vi "Get Double Message.vi"(8 "error in (no error)":errorcluster, 11 "Message Double in":refnum<class "Message Double.lvclass">) -> (0 "error out":errorcluster, 1 "Value":dbl, 2 "Name":string, 3 "Message Double out":refnum<class "Message Double.lvclass">)   [LabVIEW 2016, in "Stream Mediator.lvlib" / "Message Double.lvclass"]
doc: "--\nCopyright © 2017 Composed SystemsI All rights reserved.\n\nAuthor: Jon McBee <jon.mcbee@composed.io>\n\nThis library is provided \"AS IS\" ,WITHOUT WARRANTIES OR\nCONDITIONS OF ANY KIND, either express or implied.\n\nComposed Systems -- composed.io\n\nStream 0.0.1.1\nJon McBee - Composed Systems\nCopyright (c) 2017, Composed Systems"
uses:
  <userlib>/Composed Systems/Stream/Mediator/Classes/Message Double/Message Double.lvclass
  C:/Program Files (x86)/National Instruments/LabVIEW 2016/user.lib/Composed Systems/Stream/Mediator/Classes/Message Interface/Message Interface.lvclass
  <userlib>/Composed Systems/Stream/Mediator/Classes/Message Double/Message Double.lvclass/Message Double.ctl
  <userlib>/Composed Systems/Stream/Mediator/Classes/Message Interface/Message Interface.lvclass
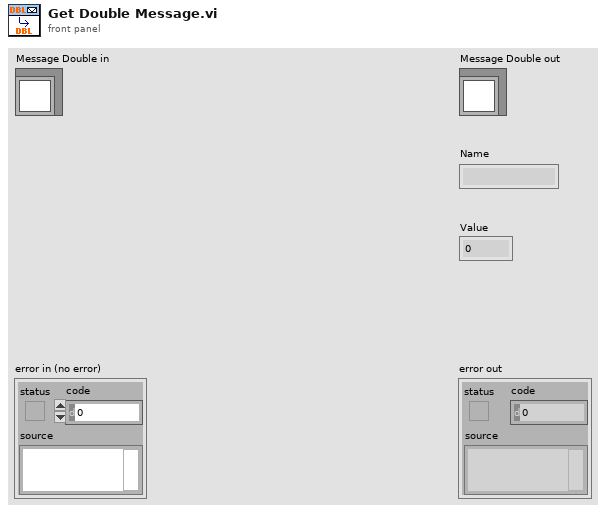
[diagram p1: front panel]
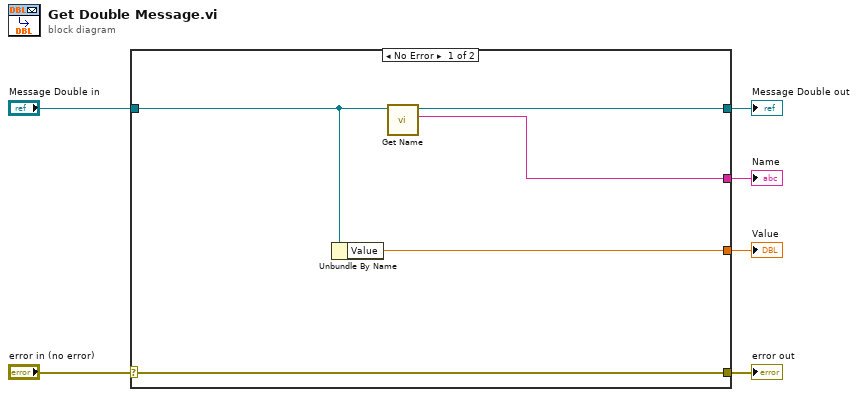
[diagram p0: block diagram]
diagram:
  n1 = case shown="No Error" "error in (no error)" {
    selector: "error in (no error)" -> [w11 w13]
    tunnel: [w11 w13] -> w5
    tunnel: [w10 w12] -> w3
    tunnel: "Message Double in" -> [w8 w12]
    tunnel: [w9 _] -> w2
    tunnel: [w7 _] -> w1
    frame No Error {
      n2 = Unbundle By Name(w8) -> ("Value"=w7:dbl)
      n3 = call <userlib>:"Get Name.vi"("Message Interface in"=w8) -> ("Name"=w9:string, "Message Interface out"=w10:refnum<class "Message Double.lvclass">)  [unwired: 8 in, 1 out]
    }
    frame Error {
    }
  }
  "error out" <- w5
  "Message Double out" <- w3
  "Name" <- w2
  "Value" <- w1
